vi "Write Config Signal.vi"(8 "error in (no error)":errorcluster, 10 "Config Signal":T1={"offset"=0.0, "square wave duty cycle (%)"=50.0, "reset signal"=FALSE, "sampling info"={"Fs"=1000.0, "#s"=1000.0}, "phase"=0.0, "signal type"=enum."Sine Wave", "amplitude"=1.0, "frequency"=10.0} {"frequency" format="%0.2p"; "amplitude" format="%0.2p"; "phase" format="%.2p"; "sampling info"."Fs" format="%.2p"; "square wave duty cycle (%)" format="%0.2f"; "offset" format="%0.2p"}, 11 "Generador in":refnum<class "Generador.lvclass">) -> (0 "error out":errorcluster, 3 "Generador out":refnum<class "Generador.lvclass">)   [LabVIEW 2020, in "Generador.lvlib" / "Generador.lvclass"]
uses:
  Generador.lvclass
  Generador.lvclass/Generador.ctl
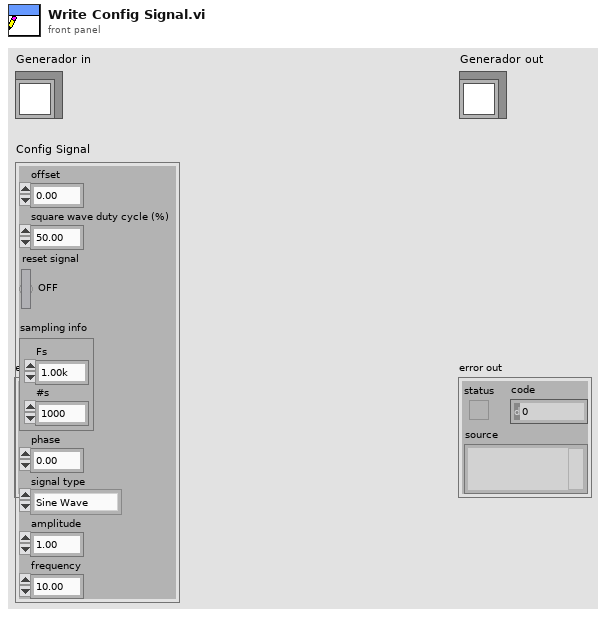
[diagram p1: front panel]
types:
  T1 = cluster{"offset":dbl, "square wave duty cycle (%)":dbl, "reset signal":bool, "sampling info":cluster{"Fs":dbl, "#s":dbl}, "phase":dbl, "signal type":enum16{"Sine Wave", "Triangle Wave", "Square Wave", "Sawtooth Wave"}, "amplitude":dbl, "frequency":dbl}
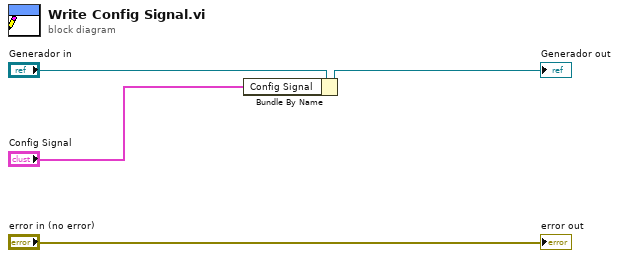
[diagram p0: block diagram]
diagram:
  n1 = Bundle By Name(cluster="Generador in", "Config Signal"="Config Signal") -> (→"Generador out":refnum<class "Generador.lvclass">)
  "error out" <- "error in (no error)"
